vi "newton_eqn.vi"(4 "dt":dbl, 6 "b1_v_init":dbl caption="body1_initial_vel", 7 "r":dbl caption="Distance bw bodies (m)", 8 "error in":errorcluster, 9 "b2_m":dbl caption="body2_mass", 10 "b1_m":dbl caption="body1_mass", 11 "b1_s0":dbl caption="body1_initial_pos") -> (0 "error out":errorcluster, 3 "b1_s1":dbl caption="body1_final_pos")   [LabVIEW 2020]
panel:
  out "F":dbl
  # "m"
  # "m"
  # "m"
  # "kg"
  # "N"
  # "kg"
  # "m/s"
  # "s"
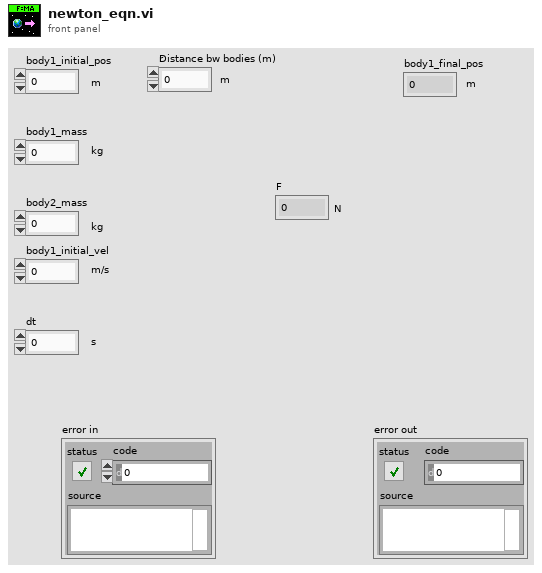
[diagram p1: front panel]
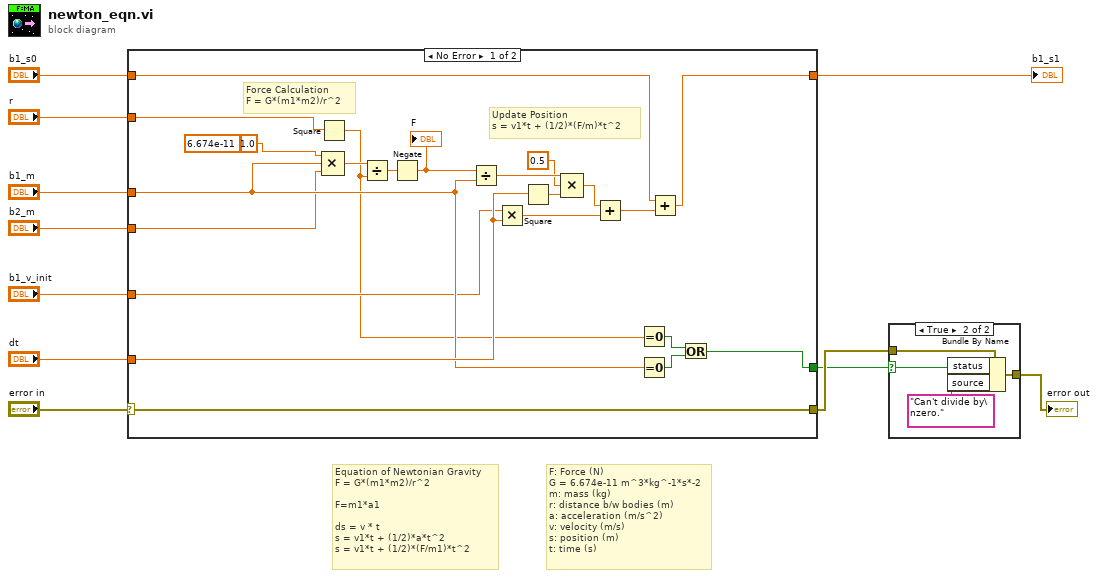
[diagram p0: block diagram]
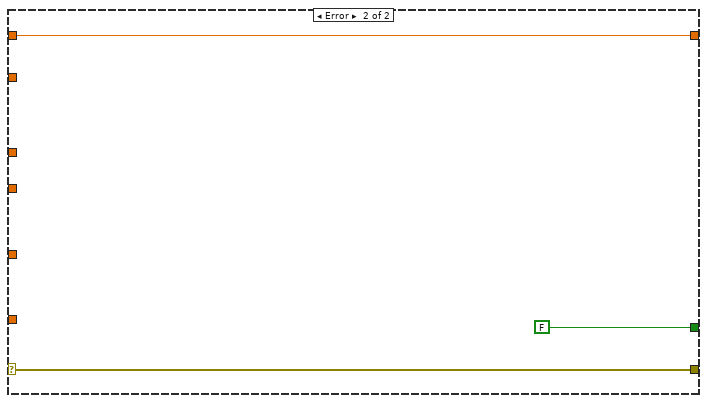
[diagram p3: hidden frame]
diagram:
  # "F: Force (N)\nG = 6.674e-11 m^3*kg^-1*s*-2 \nm: mass (kg)\nr: distance b/w bodies (m)\na: acceleration (m/s^2)\nv: velocity (m/s)\ns: position (m)\nt: time (s)"
  # "Equation of Newtonian Gravity\nF = G*(m1*m2)/r^2\n\nF=m1*a1\n\nds = v * t\ns = v1*t + (1/2)*a*t^2\ns = v1*t + (1/2)*(F/m1)*t^2"
  n1 = case shown="No Error" "error in" {
    selector: "error in" -> [w24 w36]
    tunnel: "dt" -> [w33 _]
    tunnel: [w32 w35] -> w10
    tunnel: "b1_s0" -> [w31 w35]
    tunnel: "b1_v_init" -> [w22 _]
    tunnel: "b1_m" -> [w23 _]
    tunnel: [w24 w36] -> w5
    tunnel: [w15 FALSE] -> w4
    tunnel: "r" -> [w19 _]
    tunnel: "b2_m" -> [w21 _]
    frame No Error {
      (unwired) 6.674e-11
      # "Force Calculation\nF = G*(m1*m2)/r^2"
      # "Update Position\ns = v1*t + (1/2)*(F/m)*t^2"
      n2 = Square(x=w19) -> (x^2=w16:dbl)
      n3 = Compound Arithmetic op=MULTIPLY(1.0, w23, w21) -> (w20:dbl)
      n4 = Divide(x=w20, y=w16) -> (x/y=w13:dbl)
      n5 = Negate(x=w13) -> (-x=w12:dbl)
      "F" <- w12
      n6 = Divide(x=w12, y=w23) -> (x/y=w27:dbl)
      n7 = Multiply(x=w22, y=w33) -> (x*y=w25:dbl)
      n8 = Square(x=w33) -> (x^2=w28:dbl)
      n9 = Compound Arithmetic op=MULTIPLY(w27, 0.5 ("Numeric 3"), w28) -> (w29:dbl)
      n10 = Add(x=w29, y=w25) -> (x+y=w30:dbl)
      n11 = Equal To 0?(x=w16) -> (x = 0?=w18:bool)
      n12 = Equal To 0?(x=w23) -> (x = 0?=w17:bool)
      n13 = Add(x=w31, y=w30) -> (x+y=w32:dbl)
      n14 = Or(x=w18, y=w17) -> (x .or. y?=w15:bool)
    }
    frame Error {
    }
  }
  "b1_s1" <- w10
  n15 = case shown="True" w4 {
    selector: w4 -> [_ w40]
    tunnel: w5 -> [w37 w41]
    tunnel: [w37 w38] -> w3
    frame False {
    }
    frame True {
      n16 = Bundle By Name(cluster=w41, "status"=w40, "source"="Can't divide by\nzero.") -> (w38:errorcluster)
    }
  }
  "error out" <- w3
